vi "PXI - Reserve Trigger.vi"() -> ()   [LabVIEW 2023]
doc: "This example opens a session to a PXI BACKPLANE resource and reserves trigger lines for an identified PXI system. The PXI BACKPLANE resource follows the format\n \nPXI0::?::BACKPLANE \n\nwhere ? is the number of the PXI chassis in NI MAX (Measurement & Automation Explorer). \n\n<b>Note:</b> The unreserve call executes only if the VI reserves the trigger lines successfully. Use caution when unreserving triggers, as you can remove automatic reservations made by drivers, such as NI-DAQmx, which can result in hardware damage.\n\nFor more information on PXI Timing and Triggering, refer to the KnowledgeBase at ni.com/support."
uses:
  <vilib>/Instr/_visa.llb/VISA Assert Trigger Protocol.ctl
panel:
  in  "Trigger Bus Number":i16=1
  in  "PXI Trigger Number":i16
  in  "Unreserve Trigger":bool
  in  "Stop":bool
  in  "PXI Backplane VISA resource name":refnum<visa-resource-name>
  in  "Reserve Trigger":bool
  # "Overview: Demonstrates the use of the VISA functions to reserve a trigger on a PXI backplane.\nRequirements: NI-VISA Driver, PXI device\nInstructions:\n1. Ensure the device specified by the PXI Backplane VISA resource name control is properly configured in Measurement & Automation Explorer.\n2. Run the VI.\n3. Click the Reserve Trigger and Unreserve Trigger buttons to manipulate the PXI backplane trigger.\n4. Click Stop to stop the VI."
  # "Note: This example can undo automatic trigger reservation."
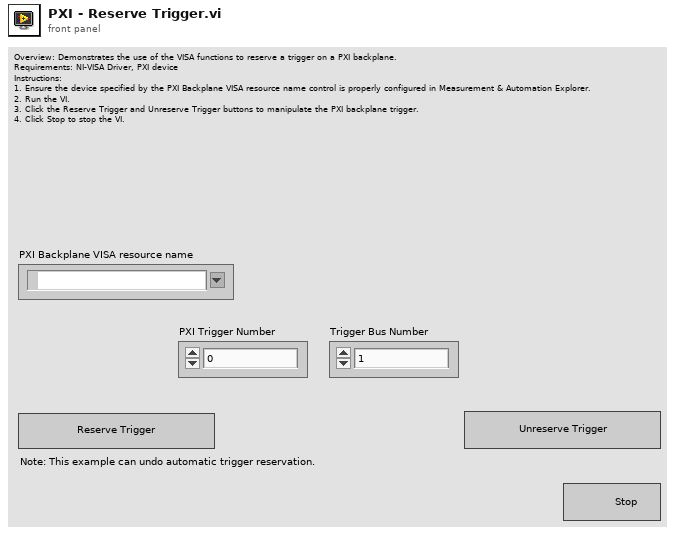
[diagram p1: front panel]
types:
  T1 = typedef "VISA Assert Trigger Protocol.ctl" = u16
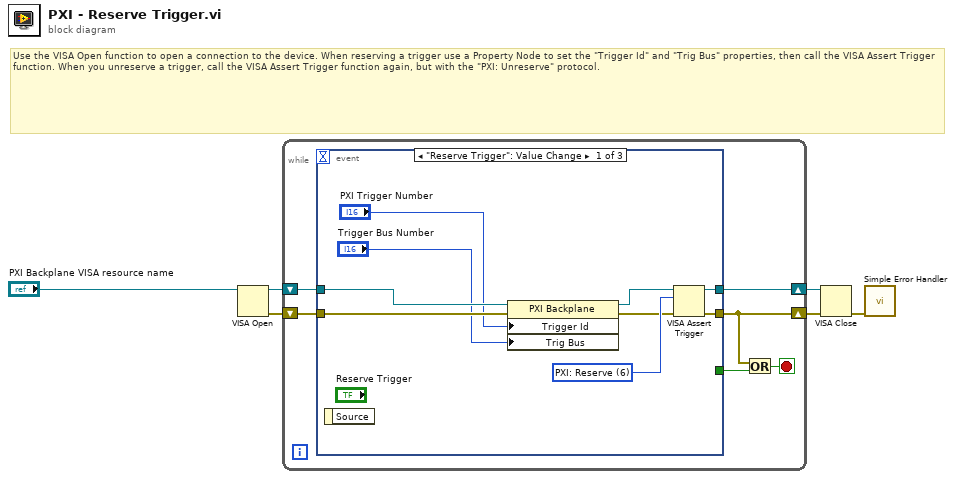
[diagram p0: block diagram]
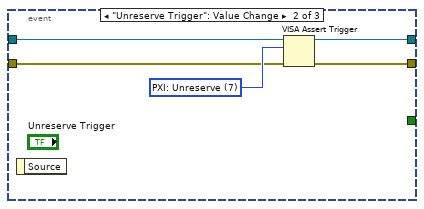
[diagram p2: hidden frame]
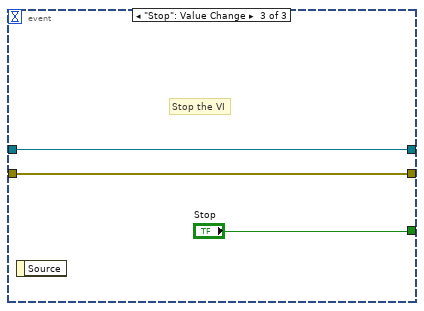
[diagram p3: hidden frame]
diagram:
  # "Use the VISA Open function to open a connection to the device. When reserving a trigger use a Property Node to set the \"Trigger Id\" and \"Trig Bus\" properties, then call the VISA Assert Trigger function. When you unreserve a trigger, call the VISA Assert Trigger function again, but with the \"PXI: Unreserve\" protocol."
  n1 = VISA Open(VISA resource name="PXI Backplane VISA resource name") -> (VISA resource name=w4:refnum<visa-resource-name>, error out=w5:errorcluster)  [unwired: 1 in, 3 out]
  n2 = while {
    shift-right: [w8] -> w3
    shift-left: w5 -> [w7]
    shift-right: [w10] -> w1
    shift-left: w4 -> [w9]
    stop <- w11 stop-if-true
    n3 = event shown="[0] \"Reserve Trigger\": Value Change" {
      selector: _ -> [_ _ _]
      dyn-events: _ -> [_ _ _]
      timeout: _ -> [_ _ _]
      tunnel: [_ _ "Stop"] -> w12
      tunnel: [w20 w22 w28] -> w8
      tunnel: w7 -> [w17 w23 w28]
      tunnel: [w21 w25 w27] -> w10
      tunnel: w9 -> [w19 w26 w27]
      event "Reserve Trigger": Value Change {
        w16 = T1 6 items=["Default"=0, "On"=1, "Off"=2, "Sync"=5, "PXI: Reserve"=6, "PXI: Unreserve"=7] ("Protocol")
        n4 = event-data() -> ()  [unwired: 2 out]
        n5 = property class="PXI Backplane"(reference=w19, error in=w17, "Trigger Id"="PXI Trigger Number", "Trig Bus"="Trigger Bus Number") -> (reference out=w18:refnum<visa-resource-name>, error out=w15:errorcluster)
        n6 = VISA Assert Trigger(8:w15, 10:w16, 11:w18) -> (0:w20:errorcluster, 3:w21:refnum<visa-resource-name>)
      }
      event "Unreserve Trigger": Value Change {
        w24 = T1 7 items=["Default"=0, "On"=1, "Off"=2, "Sync"=5, "PXI: Reserve"=6, "PXI: Unreserve"=7] ("Protocol")
        n7 = event-data() -> ()  [unwired: 2 out]
        n8 = VISA Assert Trigger(8:w23, 10:w24, 11:w26) -> (0:w22:errorcluster, 3:w25:refnum<visa-resource-name>)
      }
      event "Stop": Value Change {
        # "Stop the VI"
        n9 = event-data() -> ()  [unwired: 2 out]
      }
    }
    n10 = Or(x=w8, y=w12) -> (x .or. y?=w11:bool)
  }
  n11 = VISA Close(VISA resource name=w1, error in (no error)=w3) -> (error out=w2:errorcluster)
  n12 = call <vilib>:"Simple Error Handler.vi"("error in (no error)"=w2) -> ()  [unwired: 1 in, 8 out]
